vi "read_Pot_V0.vi"(8 "file_name":string="Pot_V0.txt") -> (2 "V0_bypass_valve":dbl, 3 "V0_run_valve":dbl)   [LabVIEW 2019]
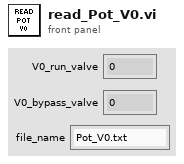
[diagram p1: front panel]
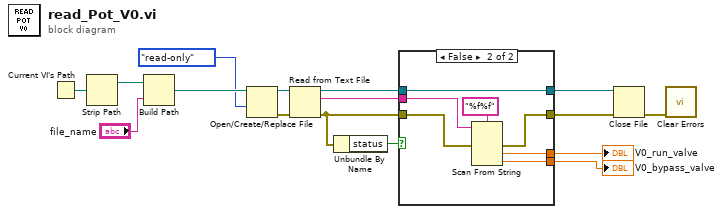
[diagram p0: block diagram]
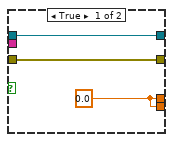
[diagram p2: hidden frame]
diagram:
  n1 = Current VI's Path() -> (path=w14:path)
  n2 = Strip Path(path=w14) -> (stripped path=w13:path)  [unwired: 1 out]
  n3 = Build Path(base path=w13, name or relative path="file_name") -> (appended path=w12:path)
  n4 = Open/Create/Replace File(file path (use dialog)=w12, access (0:read/write)=enum16{"read/write", "read-only", "write-only"}."read-only") -> (refnum out=w15:refnum<file>, error out=w9:errorcluster)  [unwired: 4 in, 1 out]
  n5 = Read from Text File(file (use dialog)=w15, error in=w9) -> (refnum out=w4:refnum<file>, text=w16:string, error out=w5:errorcluster)  [unwired: 2 in, 1 out]
  n6 = Unbundle By Name(w5) -> ("status"=w2:bool)
  n7 = case shown="False" w2 {
    tunnel: w16 -> [_ w26]
    tunnel: [w18 w24] -> w8
    tunnel: [w17 w23] -> w7
    tunnel: [w17 w22] -> w6
    tunnel: w5 -> [w18 w21]
    tunnel: w4 -> [w19 w20]
    tunnel: [w19 w20] -> w3
    frame True {
      w17 = 0.0
    }
    frame False {
      n8 = Scan From String(format string="%f%f", input string=w26, error in=w21) -> (error out=w24:errorcluster, output 1=w23:dbl, output 2=w22:dbl)  [unwired: 3 in, 2 out]
    }
  }
  "V0_run_valve" <- w7
  "V0_bypass_valve" <- w6
  n9 = Close File(refnum=w3, error in=w8) -> (error out=w1:errorcluster)  [unwired: 1 out]
  n10 = call <vilib>:"Clear Errors.vi"("error in (no error)"=w1) -> ()  [unwired: 5 in, 2 out]
